vi "CreatIP.vi"(11 "file Path":path) -> (1 "IT IP":string, 2 "Scan IP":string, 3 "IO IP":string, 4 "COM":string)   [LabVIEW 2014]
uses:
  <vilib>/Utility/file.llb/Read From Spreadsheet File (string).vi
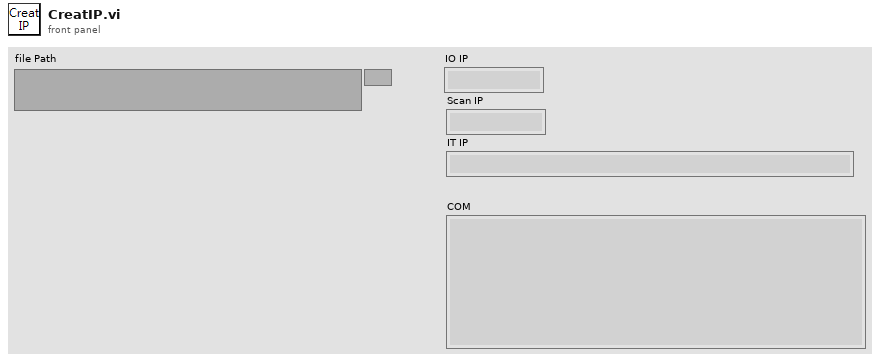
[diagram p1: front panel]
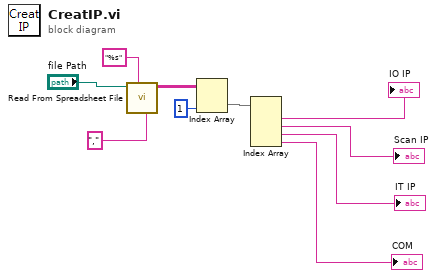
[diagram p0: block diagram]
diagram:
  n1 = call-poly <vilib>:"Read From Spreadsheet File.vi"("delimiter (\\t)"="," ("delimiter (\\t)"), "format (%s)"="%s", "file path (dialog if empty)"="file Path") -> ("all rows"=w8:string[][])  [unwired: 4 in, 4 out]
  n2 = Index Array(array=w8, index (col)=1 ("disabled index (col)")) -> (element=w6:string[])  [unwired: 1 in]
  n3 = Index Array(array=w6) -> (element #1=→"IO IP":string, element #2=→"Scan IP":string, element #3=→"IT IP":string, element #4=→"COM":string)  [unwired: 4 in]
